vi "Pkt - Get Target IP.vi"(8 "error in":errorcluster, 11 "Item Ref in":T1 format="%.0x") -> (0 "error out":errorcluster, 2 "IPAddress":string, 3 "Item Ref out":T1 format="%.0x")   [LabVIEW 2019, in "UDP-Custom-Device System Explorer.lvlib"]
uses:
  UDP-Custom-Device System Explorer.lvlib
  <vilib>/NI VeriStand/Custom Device API/Custom Device Item Ref.ctl
  NationalInstruments.VeriStand.SystemDefinitionAPI
  <vilib>/NI VeriStand/Custom Device Tools/Custom Device Utility Library/Custom Device Utility Library.lvlib
  <vilib>/NI VeriStand/Custom Device API/Custom Device API.lvlib
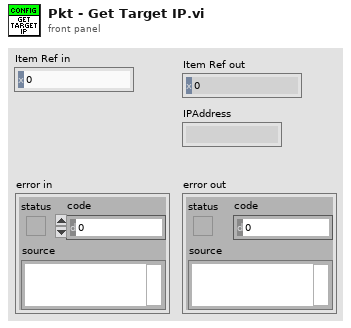
[diagram p1: front panel]
types:
  T1 = typedef "Custom Device API.lvlib/Custom Device Item Ref.ctl" = u64
  T2 = typedef "Custom Device API.lvlib/Custom Device Pointer.ctl" = refnum<k24>
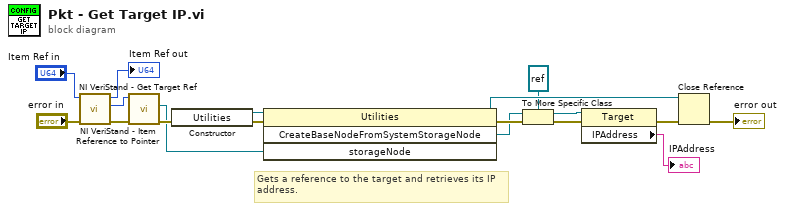
[diagram p0: block diagram]
diagram:
  # "Gets a reference to the target and retrieves its IP\naddress."
  n1 = call <vilib>:"NI VeriStand - Get Target Ref.vi"("error in"="error in", "Item Ref in"="Item Ref in") -> ("error out"=w16:errorcluster, "Target Ref"=w15:T1, "Item Ref out"=→"Item Ref out":T1)  [unwired: 6 in, 1 out]
  n2 = call <vilib>:"NI VeriStand - Item Reference to Pointer.vi"("error in (no error)"=w16, "Item Ref in"=w15) -> ("error out"=w17:errorcluster, "Node Pointer"=w14:T2)  [unwired: 6 in, 2 out]
  n3 = constructor class="Utilities"(error in=w17) -> (reference out=w6:refnum<k24>, error out=w18:errorcluster)  [unwired: 2 in, 1 out]
  n4 = invoke class="Utilities" method="CreateBaseNodeFromSystemStorageNode"(reference=w6, error in=w18, "storageNode"=w14) -> (reference out=w13:refnum<k24>, error out=w11:errorcluster, "CreateBaseNodeFromSystemStorageNode"=w7:refnum<k24>)  [unwired: 1 in, 1 out]
  n5 = To More Specific Class(target class=refnum<k24> refnum, reference=w7, error in=w11) -> (specific class reference=w9:refnum<k24>, error out=w10:errorcluster)
  n6 = property class="Target"(reference=w9, error in=w10) -> (error out=w12:errorcluster, "IPAddress"=→"IPAddress":string)  [unwired: 1 out]
  n7 = Close Reference(reference=w13, error in (no error)=w12) -> (error out=→"error out":errorcluster)
